vi "Poll Prep-Transfer Valve Control.vi"(8 "error in (no error)":errorcluster, 11 "Preparation Line in":refnum<class "Preparation Line.lvclass">) -> ()   [LabVIEW 2015, in "cRIO-Carbondioxide.lvlib" / "CO2-Actor.lvlib" / "Preparation Line.lvclass"]
uses:
  Preparation Line.lvclass
  Preparation Line.lvclass/Preparation Line.ctl
  <vilib>/ActorFramework/Actor/Actor.lvclass/Actor.ctl
  <vilib>/ActorFramework/Message Enqueuer/Message Enqueuer.lvclass/Message Enqueuer.ctl
  Preparation Line Messages/Set Transfer Valve Msg/Set Transfer Valve Msg.lvclass/Set Transfer Valve Msg.ctl
  <vilib>/ActorFramework/Actor/Read Self Enqueuer.vi
  <vilib>/ActorFramework/Message Enqueuer/Enqueue.vi
  <vilib>/ActorFramework/Message Enqueuer/Init from Existing Queue.vi
  <vilib>/ActorFramework/Message Priority Queue/Priority Enqueue.vi
  <vilib>/ActorFramework/Actor/Actor.lvclass
  <vilib>/ActorFramework/Message Enqueuer/Message Enqueuer.lvclass
  Preparation Line Messages/Set Transfer Valve Msg/Set Transfer Valve Msg.lvclass
  cRIO-CO2/cRIO-CO2.lvclass
  CO2 Actor/CO2 Actor.lvclass
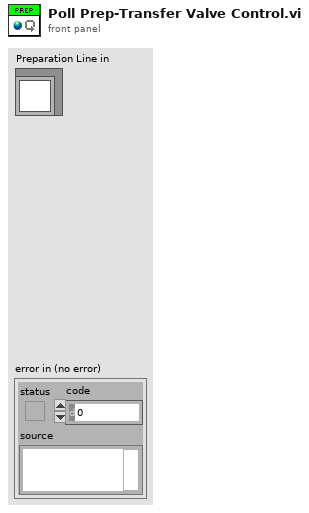
[diagram p1: front panel]
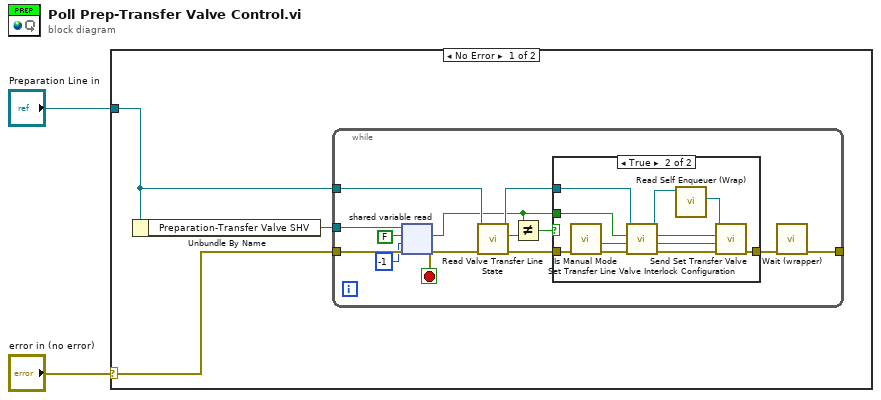
[diagram p0: block diagram]
diagram:
  n1 = case shown="No Error" "error in (no error)" {
    selector: "error in (no error)" -> [w4 _]
    tunnel: "Preparation Line in" -> [w3 _]
    frame No Error {
      n2 = Unbundle By Name(w3) -> ("Preparation-Transfer Valve SHV"=w5:refnum<k21>)
      n3 = while {
        tunnel: w5 -> [w18]
        tunnel: w4 -> [w17]
        tunnel: w3 -> [w11]
        tunnel: [w6] -> _
        stop <- w13 stop-if-true
        n4 = shared-variable-read(w18, w17, FALSE, -1 ("timeout ms")) -> (w13:errorcluster, w8:bool)  [unwired: 3 out]
        n5 = call "Read Valve Transfer Line State.vi"("error in (no error)"=w13, "Preparation Line in"=w11) -> ("error out"=w12:errorcluster, "Open?"=w9:bool, "Preparation Line out"=w10:refnum<class "Preparation Line.lvclass">)  [unwired: 6 in, 1 out]
        n6 = Not Equal?(x=w8, y=w9) -> (x != y?=w7:bool)
        n7 = case shown="True" w7 {
          tunnel: [w19 w25] -> w14
          tunnel: w12 -> [w19 w22]
          tunnel: w10 -> [_ w21]
          tunnel: w8 -> [_ w20]
          frame False {
          }
          frame True {
            n8 = call "Is Manual Mode.vi"("error in (no error)"=w22) -> ("error out"=w30:errorcluster, "Manual Mode?"=w29:bool)  [unwired: 9 in]
            n9 = call "Set Transfer Line Valve Interlock Configuration.vi"("error in (no error)"=w30, "Manual Mode (False)"=w29, "Open? (False)"=w20, "Preparation Line in"=w21) -> ("error out"=w28:errorcluster, "Interlock Chain"=w23:refnum<class "Interlock Chain.lvclass">, "Open? (False)"=w24:bool, "Preparation Line out"=w27:refnum<class "Preparation Line.lvclass">)  [unwired: 4 in]
            n10 = call "Read Self Enqueuer (Wrap).vi"("CO2 Actor in"=w27) -> ("Actor Framework:Message Enqueuer"=w26:refnum<class "Message Enqueuer.lvclass">)  [unwired: 9 in, 1 out]
            n11 = call "Send Set Transfer Valve.vi"("error in (no error)"=w28, "Interlock Chain.lvclass"=w23, "Open? (False)"=w24, "Message Enqueuer"=w26) -> ("error out"=w25:errorcluster)  [unwired: 6 in, 1 out]
          }
        }
        n12 = call "Wait (wrapper).vi"("error in (no error)"=w14) -> ("error out"=w6:errorcluster)  [unwired: 10 in]
      }
    }
    frame Error {
    }
  }
